vi "Create and Start gRPC Server.vi"(5 "Server Key File (.key)":path, 7 "Server Certificate File (.crt)":path, 8 "error in (no error)":errorcluster, 10 "Server Address":string="localhost:15882", 11 "Plugin Manager in":refnum<class "CIFPluginManager.lvclass">) -> (0 "error out":errorcluster, 3 "Plugin Manager out":refnum<class "CIFPluginManager.lvclass">)   [LabVIEW 2021, in "CIFPluginManager.lvclass"]
uses:
  CIFPluginManager.lvclass
  <vilib>/gRPC/LabVIEW gRPC Servicer/Servicer/Servicer.lvclass/Servicer.ctl
  CIFPluginManager.lvclass/CIFPluginManager.ctl
  <vilib>/gRPC/LabVIEW gRPC Servicer/Servicer/Servicer.lvclass
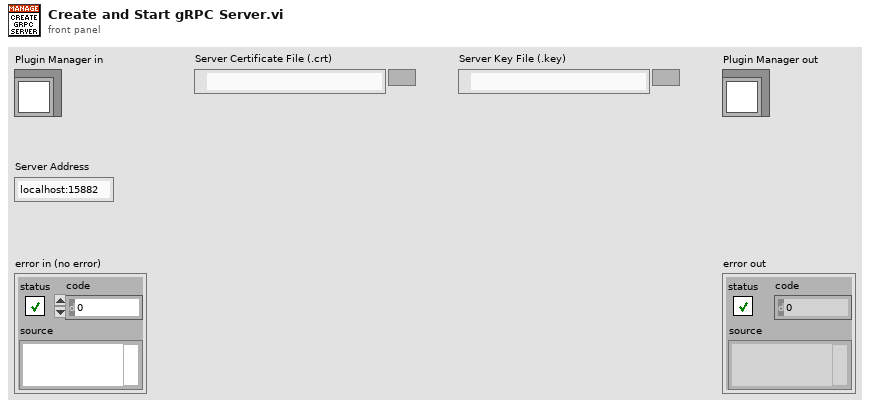
[diagram p1: front panel]
types:
  T1 = typedef "grpc-lvsupport-release.lvlib/grpcId.ctl" = u64
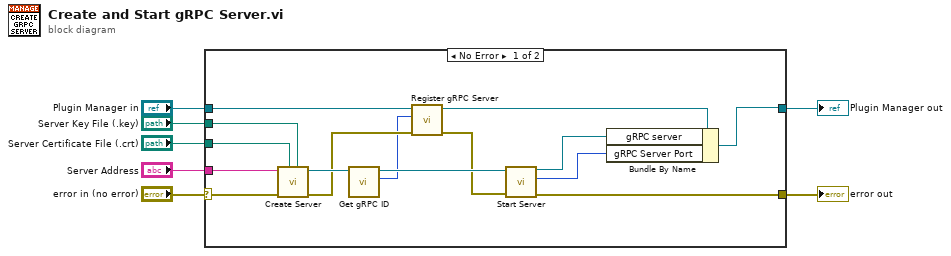
[diagram p0: block diagram]
diagram:
  n1 = case shown="No Error" "error in (no error)" {
    selector: "error in (no error)" -> [w18 w24]
    tunnel: [w17 w24] -> w2
    tunnel: [w13 w23] -> w6
    tunnel: "Plugin Manager in" -> [w11 w23]
    tunnel: "Server Certificate File (.crt)" -> [w20 _]
    tunnel: "Server Key File (.key)" -> [w19 _]
    tunnel: "Server Address" -> [w15 _]
    frame No Error {
      n2 = call <vilib>:"Create Server.vi"("Server Key File (.key)"=w19, "Server Certificate File (.crt)"=w20, "error in"=w18, "Server Address"=w15) -> ("error out"=w12:errorcluster, "gRPC server out"=w22:refnum<class "Servicer.lvclass">)  [unwired: 6 in]
      n3 = call <vilib>:"Get gRPC ID.vi"("gRPC server in"=w22) -> ("gRPC ID"=w8:T1, "gRPC server out"=w21:refnum<class "Servicer.lvclass">)  [unwired: 9 in]
      n4 = call "Register gRPC Server.vi"("error in (no error)"=w12, "gRPC ID"=w8, "Plugin Manager in"=w11) -> ("error out"=w10:errorcluster, "Plugin Manager out"=w9:refnum<class "CIFPluginManager.lvclass">)  [unwired: 7 in]
      n5 = call <vilib>:"Start Server.vi"("error in"=w10, "gRPC server in"=w21) -> ("error out"=w17:errorcluster, "Listening Port"=w16:i32, "gRPC server out"=w14:refnum<class "Servicer.lvclass">)  [unwired: 7 in]
      n6 = Bundle By Name(cluster=w9, "gRPC server"=w14, "gRPC Server Port"=w16) -> (w13:refnum<class "CIFPluginManager.lvclass">)
    }
    frame Error {
    }
  }
  "error out" <- w2
  "Plugin Manager out" <- w6
